vi "HamburgerUI.vi"() -> ()   [LabVIEW 2019]
doc: "This template is for the Queued Message Handler design pattern.\n\nThe Event Handling Loop generates messages based on user interface actions.\n\nThe Message Handling Loop processes messages generated by the Event Handling Loop, or by other messages. The messages are string values, so new messages can be added easily to the Message Cases case structure in the Message Handling Loop. Each message cluster can also provide an optional value for Message Data, which is a variant that can be converted to whatever message-specific data is required."
uses:
  controls/Hamburger UI Data.ctl
  support/Message Queue/Enqueue Message (Single).vi
  <vilib>/Utility/error.llb/Error Cluster From Error Code.vi
  <vilib>/ErrorRing/Error Ring.xnode
  support/Message Queue/Message Named Queue.lvlib
  support/User Event - Stop/User Event - Stop.lvlib
panel:
  in  "Buttons":T1
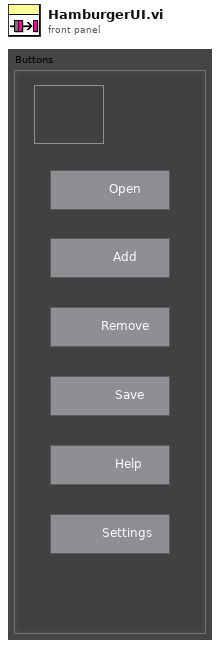
[diagram p1: front panel]
types:
  T1 = cluster{"Help":bool, "Settings":bool, "Save":bool, "Add":bool, "File Open":bool, "Remove":bool, "Cancelled":bool}
  T2 = typedef "Hamburger UI Data.ctl" = cluster{"This VI ref":refnum<vi>, "Caller ref":refnum<vi>}
  T3 = typedef "Message Named Queue.lvlib/All Message Queues.ctl" = cluster{"Main UI":refnum<queue>, "Hamburger UI":refnum<queue>}
  T4 = enum32{"Invalid", "Standard", "Closed", "Hidden", "Minimized", "Maximized"}
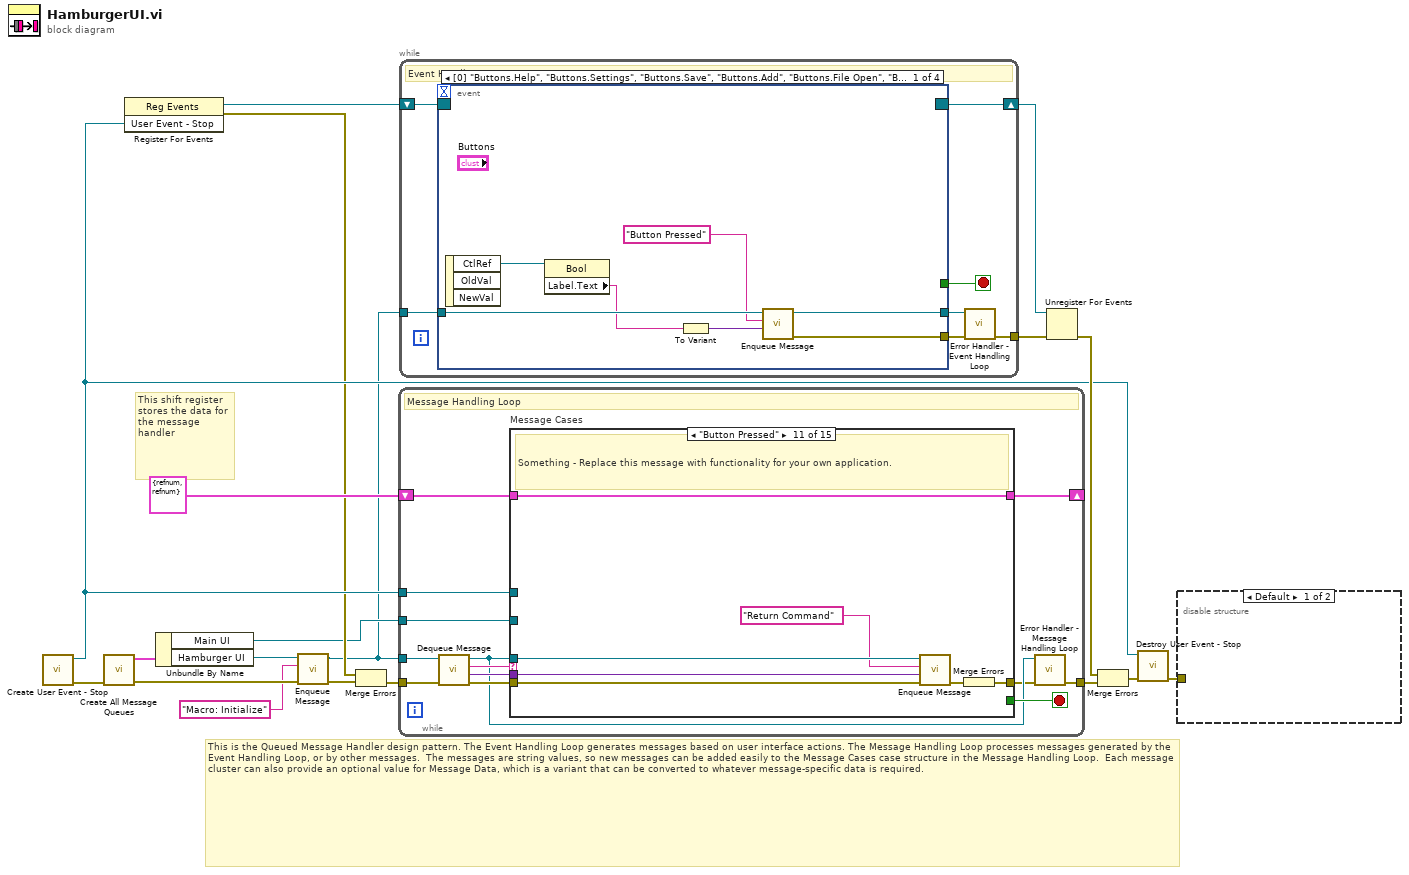
[diagram p0: block diagram]
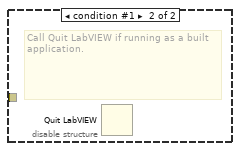
[diagram p2: hidden frame]
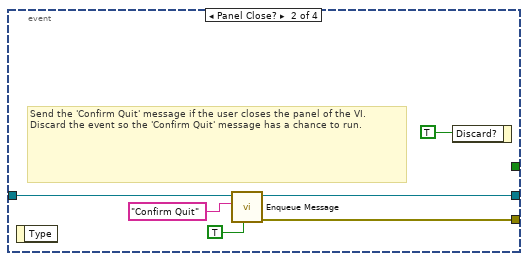
[diagram p3: hidden frame]
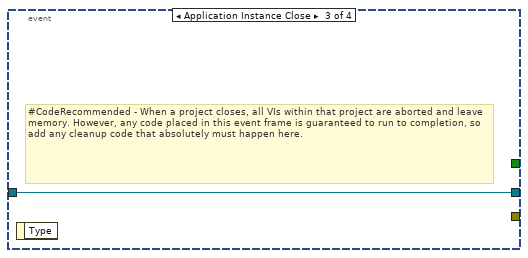
[diagram p4: hidden frame]
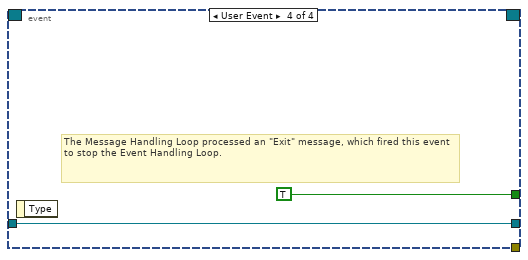
[diagram p5: hidden frame]
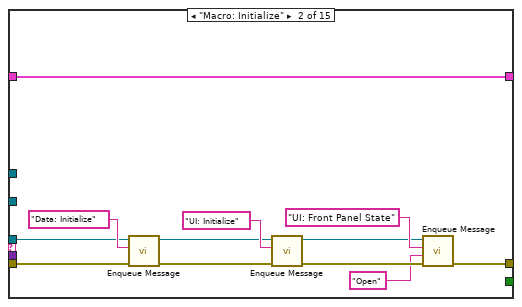
[diagram p7: hidden frame]
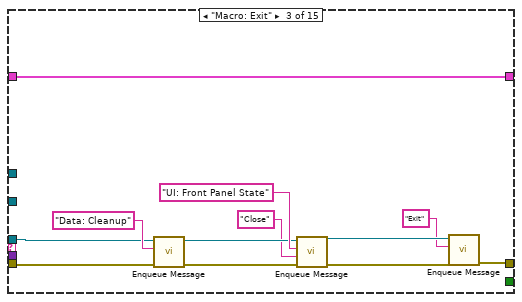
[diagram p8: hidden frame]
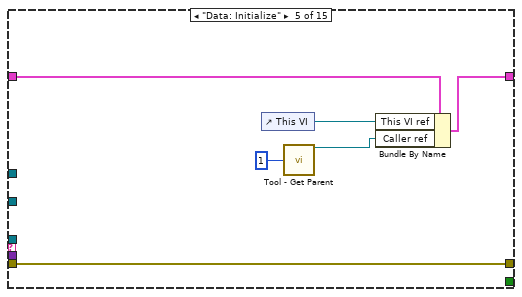
[diagram p10: hidden frame]
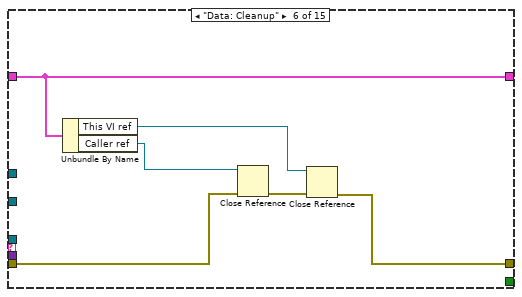
[diagram p11: hidden frame]
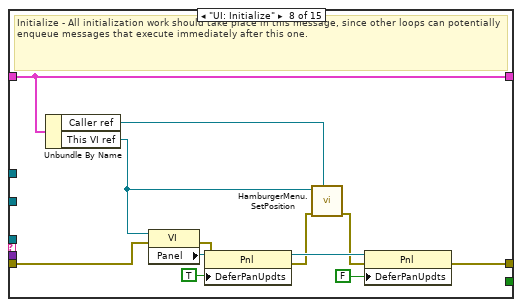
[diagram p13: hidden frame]
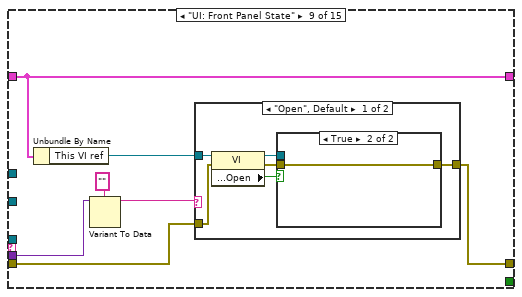
[diagram p14: hidden frame]
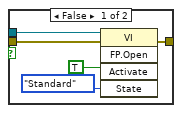
[diagram p15: hidden frame]
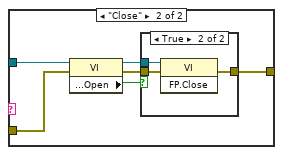
[diagram p16: hidden frame]
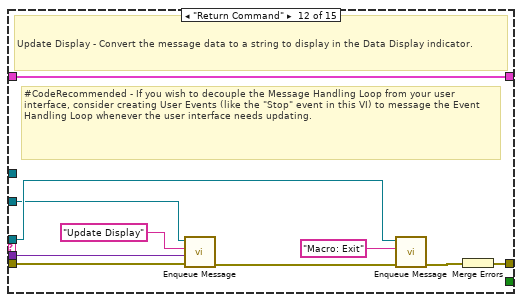
[diagram p19: hidden frame]
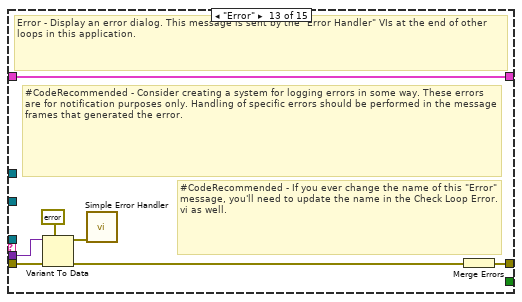
[diagram p20: hidden frame]
diagram:
  # "This is the Queued Message Handler design pattern. The Event Handling Loop generates messages based on user interface actions. The Message Handling Loop processes messages generated by the Event Handling Loop, or by other messages.  The messages are string values, so new messages can be added easily to the Message Cases case structure in the Message Handling Loop.  Each message cluster can also provide an optional value for Message Data, which is a variant that can be converted to whatever message-specific data is required."
  # "This shift register stores the data for the message handler"
  n1 = call "Create User Event - Stop.vi"() -> ("error out"=w17:errorcluster, "User Event - Stop"=w9:refnum<user-event>)  [unwired: 10 in]
  n2 = call "Create All Message Queues.vi"("error in (no error)"=w17) -> ("error out"=w3:errorcluster, "Message Queues out"=w19:T3)  [unwired: 9 in]
  n3 = register-events(w9) -> (reference out=w10:refnum<event-registration>, error out=w7:errorcluster)  [unwired: 2 in]
  n4 = Unbundle By Name(w19) -> ("Main UI"=w6:refnum<queue>, "Hamburger UI"=w5:refnum<queue>)
  n5 = call-poly "Enqueue Message.vi"("error in (no error)"=w3, "Message"="Macro: Initialize", "Message Queue"=w5) -> ("error out"=w4:errorcluster, "dup Message Queue"=w1:refnum<queue>)  [unwired: 7 in]
  n6 = Merge Errors(w7, w4) -> (w8:errorcluster)
  n7 = while {
    tunnel: w1 -> [w24]
    shift-right: [w31] -> _
    shift-left: T2 {"This VI ref"=refnum, "Caller ref"=refnum} ("Data Cluster") -> [w32]
    tunnel: w9 -> [w29]
    tunnel: w8 -> [w28]
    tunnel: [w22] -> w18
    tunnel: w6 -> [w20]
    stop <- w30 stop-if-true
    # "Message Handling Loop"
    n8 = call "Dequeue Message.vi"("error in (no error)"=w28, "Message Queue"=w24) -> ("error out"=w27:errorcluster, "Message Data"=w25:variant, "Message"=w26:string, "dup Message Queue"=w23:refnum<queue>)  [unwired: 6 in]
    n9 = case "Message Cases" shown="\"Button Pressed\"" w26 {
      selector: w26 -> [_ _ _ _ _ _ _ _ _ _ _ _ _ _ w153]
      tunnel: w23 -> [_ w41 w52 _ _ _ _ _ _ _ w121 w131 _ w152 _]
      tunnel: w27 -> [w34 w43 w53 w60 w66 w71 w74 w82 w92 w117 w123 w129 w141 w145 _]
      tunnel: [w34 w38 w49 w60 w66 w69 w74 w81 w93 w117 w124 w133 w135 w148 w154] -> w21
      tunnel: w32 -> [w33 w46 w58 w59 w65 w72 w73 w79 w91 w116 w119 w134 w140 w151 w155]
      tunnel: [w33 w46 w58 w59 w64 w72 w73 w79 w91 w116 w119 w134 w140 w151 w155] -> w31
      tunnel: [_ _ _ _ _ _ _ _ _ _ _ _ _ TRUE _] -> w30
      tunnel: w25 -> [_ _ _ _ _ _ _ _ w87 _ w118 w125 w139 w142 _]
      tunnel: w29 -> [_ _ _ _ _ _ _ _ _ _ _ _ _ w147 _]
      tunnel: w20 -> [_ _ _ _ _ _ _ _ _ _ _ w127 _ _ _]
      frame "---------Macro---------" {
      }
      frame "Macro: Initialize" {
        n10 = call-poly "Enqueue Message.vi"("error in (no error)"=w43, "Message"="Data: Initialize", "Message Queue"=w41) -> ("error out"=w42:errorcluster, "dup Message Queue"=w40:refnum<queue>)  [unwired: 7 in]
        n11 = call-poly "Enqueue Message.vi"("error in (no error)"=w42, "Message"="UI: Initialize", "Message Queue"=w40) -> ("error out"=w39:errorcluster, "dup Message Queue"=w36:refnum<queue>)  [unwired: 7 in]
        n12 = call-poly "Enqueue Message.vi"("error in (no error)"=w39, "Message Data"="Open" ("Message"), "Message"="UI: Front Panel State", "Message Queue"=w36) -> ("error out"=w38:errorcluster)  [unwired: 6 in, 1 out]
      }
      frame "Macro: Exit" {
        n13 = call-poly "Enqueue Message.vi"("error in (no error)"=w53, "Message"="Data: Cleanup", "Message Queue"=w52) -> ("error out"=w55:errorcluster, "dup Message Queue"=w54:refnum<queue>)  [unwired: 7 in]
        n14 = call-poly "Enqueue Message.vi"("error in (no error)"=w55, "Message Data"="Close" ("Message"), "Message"="UI: Front Panel State", "Message Queue"=w54) -> ("error out"=w50:errorcluster, "dup Message Queue"=w48:refnum<queue>)  [unwired: 6 in]
        n15 = call-poly "Enqueue Message.vi"("error in (no error)"=w50, "Message"="Exit", "Message Queue"=w48) -> ("error out"=w49:errorcluster)  [unwired: 7 in, 1 out]
      }
      frame "----------Data----------" {
      }
      frame "Data: Initialize" {
        n16 = control-ref of="This VI"() -> (w63:refnum<vi>)
        n17 = call "Tool - Get Parent.vi"("Generations Back (1:parent)"=1) -> ("VI Refnum"=w61:refnum<vi>)  [unwired: 16 in, 2 out]
        n18 = Bundle By Name(cluster=w65, "This VI ref"=w63, "Caller ref"=w61) -> (w64:T2)
      }
      frame "Data: Cleanup" {
        n19 = Unbundle By Name(w72) -> ("This VI ref"=w67:refnum<vi>, "Caller ref"=w68:refnum<vi>)
        n20 = Close Reference(reference=w68, error in (no error)=w71) -> (error out=w70:errorcluster)
        n21 = Close Reference(reference=w67, error in (no error)=w70) -> (error out=w69:errorcluster)
      }
      frame "-----------UI-----------" {
      }
      frame "UI: Initialize" {
        # "Initialize - All initialization work should take place in this message, since other loops can potentially enqueue messages that execute immediately after this one."
        n22 = Unbundle By Name(w79) -> ("Caller ref"=w78:refnum<vi>, "This VI ref"=w77:refnum<vi>)
        n23 = property class="VI"(reference=w77, error in=w82) -> (error out=w85:errorcluster, "Panel"=w84:refnum<vi>)  [unwired: 1 out]
        n24 = property class="Pnl"(reference=w84, error in=w85, "DeferPanUpdts"=TRUE ("defer panel updates")) -> (reference out=w80:refnum<vi>, error out=w76:errorcluster)
        n25 = call "HamburgerMenu.SetPosition.vi"("Caller VI Refnum"=w78, "error in (no error)"=w76, "Current VI Refnum"=w77) -> ("error out"=w75:errorcluster)  [unwired: 7 in, 1 out]
        n26 = property class="Pnl"(reference=w80, error in=w75, "DeferPanUpdts"=FALSE ("Defer Panel Updates")) -> (error out=w81:errorcluster)  [unwired: 1 out]
      }
      frame "UI: Front Panel State" {
        n27 = Unbundle By Name(w91) -> ("This VI ref"=w90:refnum<vi>)
        n28 = Variant To Data(type="", Variant=w87) -> (data=w88:string)  [unwired: 1 in, 1 out]
        n29 = case shown="\"Open\", Default" w88 {
          tunnel: w92 -> [w97 w110]
          tunnel: [w99 w111] -> w93
          tunnel: w90 -> [w98 w108]
          frame "Open", Default {
            n30 = property class="VI"(reference=w98, error in=w97) -> (reference out=w95:refnum<vi>, error out=w96:errorcluster, "Front Panel.Open"=w94:bool)
            n31 = case shown="True" w94 {
              tunnel: [w102 w105] -> w99
              tunnel: w96 -> [w101 w105]
              tunnel: w95 -> [w100 _]
              frame False {
                n32 = invoke class="VI" method="FP.Open"(reference=w100, error in=w101, "Activate"=TRUE, "State"=T4."Standard") -> (error out=w102:errorcluster)  [unwired: 1 in, 4 out]
              }
              frame True {
              }
            }
          }
          frame "Close" {
            n33 = property class="VI"(reference=w108, error in=w110) -> (reference out=w107:refnum<vi>, error out=w109:errorcluster, "Front Panel.Open"=w106:bool)
            n34 = case shown="True" w106 {
              tunnel: [w112 w115] -> w111
              tunnel: w109 -> [w112 w114]
              tunnel: w107 -> [_ w113]
              frame False {
              }
              frame True {
                n35 = invoke class="VI" method="FP.Close"(reference=w113, error in=w114) -> (error out=w115:errorcluster)  [unwired: 1 in, 2 out]
              }
            }
          }
        }
      }
      frame "----------Core----------" {
      }
      frame "Button Pressed" {
        # "Something - Replace this message with functionality for your own application."
        n36 = call-poly "Enqueue Message.vi"("error in (no error)"=w123, "Message Data"=w118, "Message"="Return Command", "Message Queue"=w121) -> ("error out"=w122:errorcluster)  [unwired: 6 in, 1 out]
        n37 = Merge Errors(w122) -> (w124:errorcluster)
      }
      frame "Return Command" {
        # "#CodeRecommended - If you wish to decouple the Message Handling Loop from your user interface, consider creating User Events (like the \"Stop\" event in this VI) to message the Event Handling Loop whenever the user interface needs updating."
        # "Update Display - Convert the message data to a string to display in the Data Display indicator."
        n38 = call-poly "Enqueue Message.vi"("error in (no error)"=w129, "Message Data"=w125, "Message"="Update Display", "Message Queue"=w127) -> ("error out"=w128:errorcluster)  [unwired: 6 in, 1 out]
        n39 = call-poly "Enqueue Message.vi"("error in (no error)"=w128, "Message"="Macro: Exit", "Message Queue"=w131) -> ("error out"=w132:errorcluster)  [unwired: 7 in, 1 out]
        n40 = Merge Errors(w132) -> (w133:errorcluster)
      }
      frame "Error" {
        # "#CodeRecommended - If you ever change the name of this \"Error\" message, you'll need to update the name in the Check Loop Error.vi as well."
        # "#CodeRecommended - Consider creating a system for logging errors in some way. These errors are for notification purposes only. Handling of specific errors should be performed in the message frames that generated the error."
        # "Error - Display an error dialog. This message is sent by the \"Error Handler\" VIs at the end of other loops in this application."
        n41 = Variant To Data(error in=w141, type=errorcluster {"status"=FALSE, "code"=0, "source"=""} ("error constant"), Variant=w139) -> (data=w137:errorcluster, error out=w136:errorcluster)
        n42 = call <vilib>:"Simple Error Handler.vi"("error in (no error)"=w137) -> ()  [unwired: 4 in, 5 out]
        n43 = Merge Errors(w136) -> (w135:errorcluster)
      }
      frame "Exit" {
        # "Stop the VI"
        # "Release the message queue reference"
        # "#CodeNeeded - Add any required cleanup code here. Note that if 'Exit' was called as a result of an error, an error dialog will be displayed. Add any custom error handling for an 'Exit' condition here as well."
        # "Exit - Exit the application."
        n44 = Variant To Data(type=errorcluster {"status"=FALSE, "code"=0, "source"=""} ("error constant"), Variant=w142) -> (data=w143:errorcluster)  [unwired: 1 in, 1 out]
        n45 = call <vilib>:"Simple Error Handler.vi"("error in (no error)"=w143) -> ()  [unwired: 4 in, 5 out]
        n46 = call "Fire User Event - Stop.vi"("User Event - Stop"=w147) -> ("error out"=w146:errorcluster)  [unwired: 10 in]
        n47 = Release Queue(queue=w152, error in (no error)=w145) -> (error out=w149:errorcluster)  [unwired: 1 in, 2 out]
        n48 = Merge Errors(w146, w149) -> (w148:errorcluster)
      }
      frame Default {
        # "'Default' case only runs if there is a message that isn't defined in any of the other cases.  Output a programming error."
        n49 = xnode "Error Ring"("parameter 0"=w153) -> ("error out"=w154:errorcluster)
      }
    }
    n50 = call "Error Handler - Message Handling Loop.vi"("error in (no error)"=w21, "Message Queue"=w23) -> ("dup error in"=w22:errorcluster)  [unwired: 8 in, 1 out]
  }
  n51 = while {
    tunnel: w1 -> [w169]
    shift-right: [w167] -> w14
    shift-left: w10 -> [w168]
    tunnel: [w163] -> w11
    stop <- w165 stop-if-true
    # "Event Handling Loop"
    n52 = event shown="[0] \"Buttons.Help\", \"Buttons.Settings\", \"Buttons.Save\", \"Buttons.Add\", \"Buttons.File Open\", \"Buttons.Remove\", \"Buttons.Cancelled\": Value Change" {
      selector: w168 -> [_ _ _ _]
      dyn-events: [_ _ _ _] -> w167
      timeout: _ -> [_ _ _ _]
      tunnel: [_ _ _ TRUE ("Discard?")] -> w165
      tunnel: w169 -> [w176 w181 w183 w185]
      tunnel: [w173 w180 _ _] -> w166
      tunnel: [w175 w179 w183 w185] -> w164
      event "Buttons.Help", "Buttons.Settings", "Buttons.Save", "Buttons.Add", "Buttons.File Open", "Buttons.Remove", "Buttons.Cancelled": Value Change {
        n53 = event-data() -> ("CtlRef"=w172:refnum<vi>)  [unwired: 1 in, 2 out]
        n54 = property class="Bool"(reference=w172) -> ("Label.Text"=w171:string)  [unwired: 1 in, 2 out]
        n55 = To Variant(anything=w171) -> (Variant=w170:variant)
        n56 = call-poly "Enqueue Message.vi"("Message Data"=w170, "Message"="Button Pressed", "Message Queue"=w176) -> ("error out"=w173:errorcluster, "dup Message Queue"=w175:refnum<queue>)  [unwired: 7 in]
      }
      event Panel Close? {
        # "Send the 'Confirm Quit' message if the user closes the panel of the VI. Discard the event so the 'Confirm Quit' message has a chance to run."
        n57 = event-data() -> ()  [unwired: 1 in, 1 out]
        n58 = call-poly "Enqueue Message.vi"("Priority Message? (F)"=TRUE, "Message"="Confirm Quit", "Message Queue"=w181) -> ("error out"=w180:errorcluster, "dup Message Queue"=w179:refnum<queue>)  [unwired: 7 in]
        n59 = event-data("Discard?"=TRUE) -> ()  [unwired: 1 in, 1 out]
      }
      event Application Instance Close {
        # "#CodeRecommended - When a project closes, all VIs within that project are aborted and leave memory. However, any code placed in this event frame is guaranteed to run to completion, so add any cleanup code that absolutely must happen here."
        n60 = event-data() -> ()  [unwired: 1 in, 1 out]
      }
      event User Event {
        # "The Message Handling Loop processed an \"Exit\" message, which fired this event to stop the Event Handling Loop."
        n61 = event-data() -> ()  [unwired: 1 in, 1 out]
      }
    }
    n62 = call "Error Handler - Event Handling Loop.vi"("error in (no error)"=w166, "Message Queue"=w164) -> ("dup error in"=w163:errorcluster)  [unwired: 8 in, 1 out]
  }
  n63 = Unregister For Events(event registration refnum=w14, error in=w11) -> (error out=w15:errorcluster)
  n64 = Merge Errors(w15, w18) -> (w16:errorcluster)
  n65 = call "Destroy User Event - Stop.vi"("error in (no error)"=w16, "User Event - Stop"=w9) -> ("error out"=w12:errorcluster)  [unwired: 9 in]
  n66 = disable-structure shown="Default" {
    disable-tunnel: w12 -> [_ _]
    frame condition #0 (active) {
    }
    frame condition #1 {
      # "Call Quit LabVIEW if running as a built application."
      n67 = Quit LabVIEW() -> ()  [unwired: 1 in]
    }
  }
